vi "Unset Busy Indicator.vi"(11 "error in (no error)":errorcluster) -> (3 "error out":errorcluster)   [LabVIEW 2023]
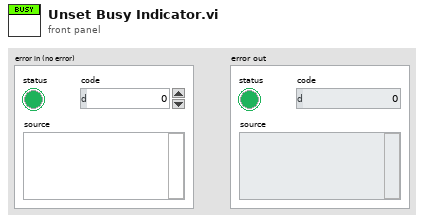
[diagram p1: front panel]
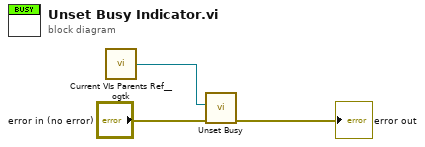
[diagram p0: block diagram]
diagram:
  n1 = call <userlib>:"Current VIs Parents Ref__ogtk.vi"() -> ("Calling VI's Reference"=w1:refnum<vi>)  [unwired: 2 in]
  n2 = call <vilib>:"Unset Busy.vi"("error in (no error)"="error in (no error)", "VI reference (current VI)"=w1) -> ("error out"=→"error out":errorcluster)  [unwired: 9 in]
